vi "Initialize.vi"(8 "error in (no error)":errorcluster, 9 "Rate":dbl, 10 "Number Of Samples Per Channel":i32) -> (0 "error out":errorcluster, 3 "Analog Input out":refnum<class "Analog Input.lvclass">)   [LabVIEW 2021, in "Analog Input.lvclass"]
uses:
  Analog Input.lvclass
  Analog Input.lvclass/Analog Input.ctl
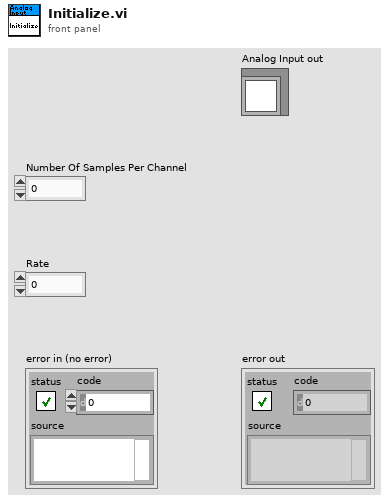
[diagram p1: front panel]
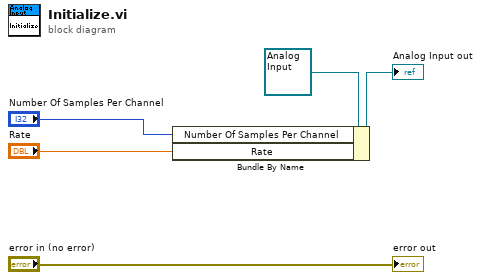
[diagram p0: block diagram]
diagram:
  n1 = Bundle By Name(cluster=refnum<class "Analog Input.lvclass"> refnum ("Input in"), "Number Of Samples Per Channel"="Number Of Samples Per Channel", "Rate"="Rate") -> (→"Analog Input out":refnum<class "Analog Input.lvclass">)
  "error out" <- "error in (no error)"
